vi "Serial Write and Read on Two Ports 4.0.vi"(10 "VISA Resource (write)":refnum<visa-resource-name>="COM5", 11 "Write String":string="DPOS=5000") -> (3 "Read String":string="EPOS=2\n")   [LabVIEW 2019]
doc: "This example opens two VISA resources and configures one COM port to perform a write operation and the other COM port to perform a read operation. This VI will wait until the specified number of bytes is received at the port or until a termination character is read.\n\nThis example allows you perform diagnostic tests on your ports. You can use this example to perform a wrap-back test. Both serial ports must have the same basic configuration parameters. You can connect two of the ports using a null modem cable, which effectively connects one port's RX lines to the other port's TX lines. If you use a straight-through cable, one port's RX lines will be connected to the other port's RX lines, and you cannot communicate between the two ports."
uses:
  Program Files (x86)/National Instruments/LabVIEW 2019/instr.lib/LPT/LPT-GUI-MIC-ver 4 Randy Folder/examples/Instrument IO/Serial/support/Serial - Settings.ctl
  <vilib>/Instr/_visa.llb/VISA Configure Serial Port (Instr).vi
panel:
  in  "Serial Settings (read)":T1={"baud rate"=9600, "data bits"=8, "parity"=enum."None", "stop bits"=10, "flow control"=0} {"flow control" items=["None"=0, "XON/XOFF"=1, "RTS/CTS"=2, "DTR/DSR"=4]; "stop bits" items=["1.0"=10, "1.5"=15, "2.0"=20]; "data bits" min=5 max=8 step=1; "baud rate" items=["75"=75, "110"=110, "134"=134, "150"=150, "300"=300, "600"=600, "1200"=1200, "1800"=1800, "2400"=2400, "4800"=4800, "7200"=7200, "9600"=9600, "14400"=14400, "19200"=19200, "28800"=28800, "38400"=38400, "56000"=56000, "57600"=57600, "115200"=115200, "128000"=128000, "230400"=230400]}
  in  "Serial Settings (write)":T1={"baud rate"=9600, "data bits"=8, "parity"=enum."None", "stop bits"=10, "flow control"=0} {"flow control" items=["None"=0, "XON/XOFF"=1, "RTS/CTS"=2, "DTR/DSR"=4]; "stop bits" items=["1.0"=10, "1.5"=15, "2.0"=20]; "data bits" min=5 max=8 step=1; "baud rate" items=["75"=75, "110"=110, "134"=134, "150"=150, "300"=300, "600"=600, "1200"=1200, "1800"=1800, "2400"=2400, "4800"=4800, "7200"=7200, "9600"=9600, "14400"=14400, "19200"=19200, "28800"=28800, "38400"=38400, "56000"=56000, "57600"=57600, "115200"=115200, "128000"=128000, "230400"=230400]}
  out "bytes read":u32=7
  out "VISA Resource (read)":refnum<visa-resource-name>="COM5"
  out "bytes written":u32=9
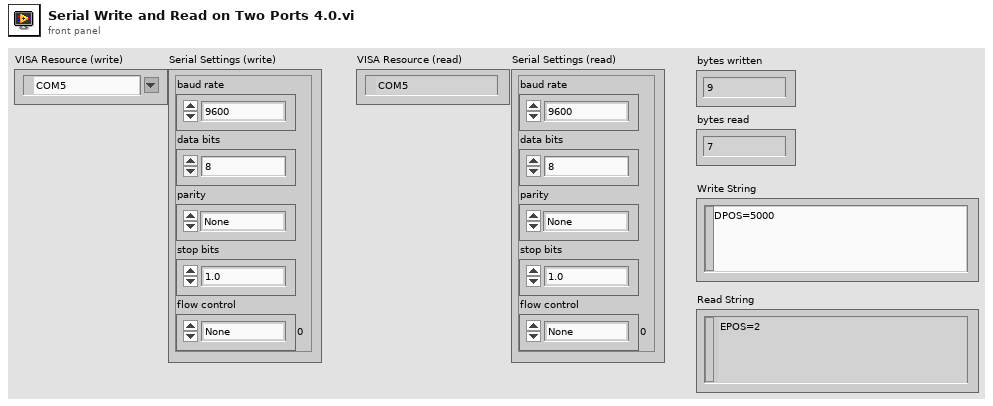
[diagram p1: front panel]
types:
  T1 = typedef "Serial - Settings.ctl" = cluster{"baud rate":u32, "data bits":u16, "parity":enum16{"None", "Odd", "Even", "Mark", "Space"}, "stop bits":u16, "flow control":u16}
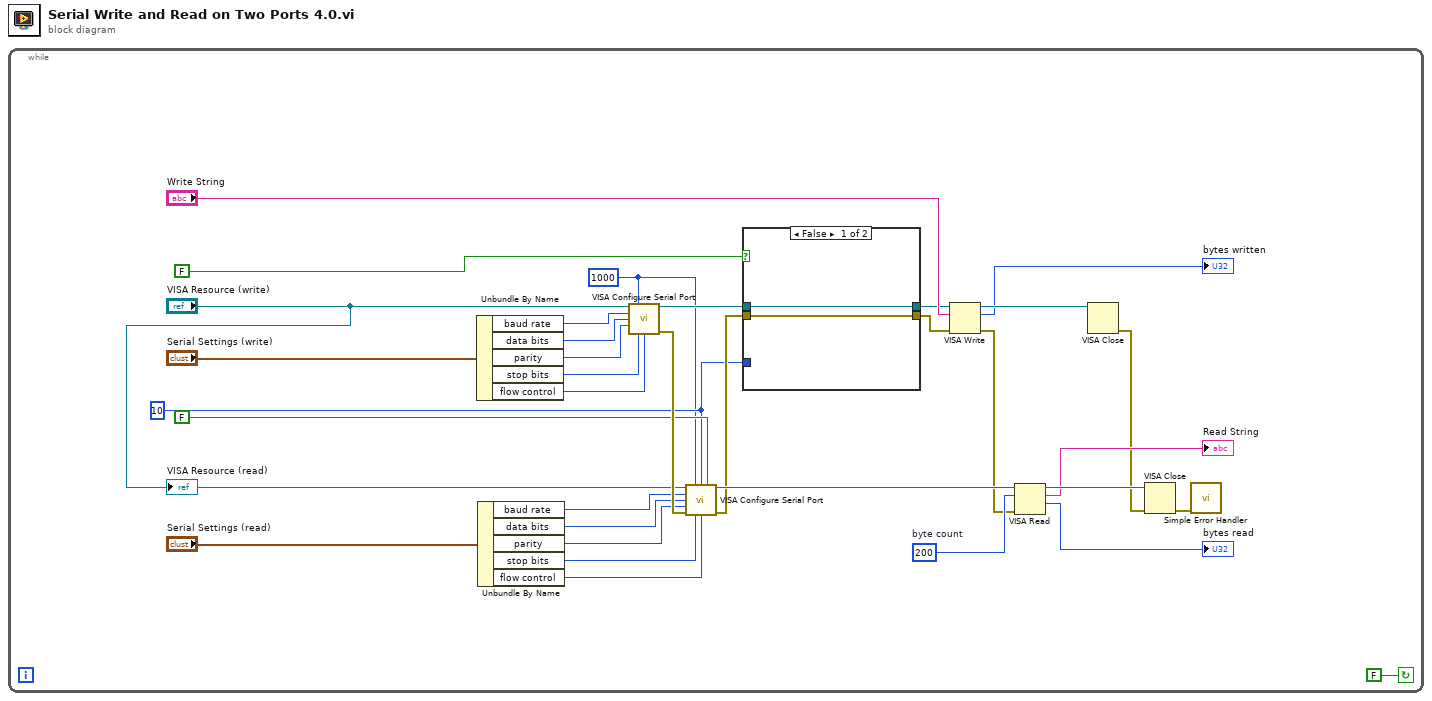
[diagram p0: block diagram]
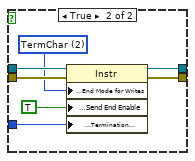
[diagram p2: hidden frame]
diagram:
  n1 = while {
    stop <- FALSE continue-if-true
    w4 = u8 10 ("Termination Character")
    w3 = u32 1000 ("timeout (10sec)")
    w29 = u32 200  # byte count
    n2 = Unbundle By Name("Serial Settings (write)") -> ("baud rate"=w22:u32, "data bits"=w21:u16, "parity"=w20:enum16{"None", "Odd", "Even", "Mark", "Space"}, "stop bits"=w19:u16, "flow control"=w18:u16)
    n3 = Unbundle By Name("Serial Settings (read)") -> ("baud rate"=w16:u32, "data bits"=w15:u16, "parity"=w14:enum16{"None", "Odd", "Even", "Mark", "Space"}, "stop bits"=w13:u16, "flow control"=w12:u16)
    n4 = call-poly "VISA Configure Serial Port"("VISA resource name"="VISA Resource (write)", "timeout (10sec)"=w3, "baud rate (9600)"=w22, "data bits (8)"=w21, "parity (0:none)"=w20, "stop bits (10: 1 bit)"=w19, "flow control (0:none)"=w18) -> ("VISA resource name out"=w9:refnum<visa-resource-name>, "error out"=w27:errorcluster)  [unwired: 2 in, 5 out]
    n5 = call-poly "VISA Configure Serial Port"("VISA resource name"="VISA Resource (write)", "timeout (10sec)"=w3, "termination char\n(0xA = '\\n' = LF)"=w4, "Enable Termination\nChar (T)"=FALSE ("End Read on Termination Character?"), "baud rate (9600)"=w16, "data bits (8)"=w15, "parity (0:none)"=w14, "error in (no error)"=w27, "stop bits (10: 1 bit)"=w13, "flow control (0:none)"=w12) -> ("VISA resource name out"=w33:refnum<visa-resource-name>, "error out"=w7:errorcluster)  [unwired: 4 out]
    n6 = case shown="False" FALSE ("End Write on Termination Character?") {
      tunnel: w9 -> [w35 w43]
      tunnel: w7 -> [w36 w42]
      tunnel: [w35 w41] -> w8
      tunnel: [w36 w40] -> w6
      tunnel: w4 -> [_ w38]
      frame False {
      }
      frame True {
        w39 = u16 2 items=["None", "LastBit", "TermChar", "Break"] ("Serial Settings:Serial End Mode for Writes")
        n7 = property class="Instr"(reference=w43, error in=w42, "Serial Settings:End Mode for Writes"=w39, "Message Based Settings:Send End Enable"=TRUE, "Message Based Settings:Termination Character"=w38) -> (reference out=w41:refnum<visa-resource-name>, error out=w40:errorcluster)
      }
    }
    n8 = VISA Write(VISA resource name=w8, write buffer="Write String", error in (no error)=w6) -> (VISA resource name out=w34:refnum<visa-resource-name>, return count=→"bytes written":u32, error out=w26:errorcluster)
    n9 = VISA Read(VISA resource name=w33, byte count=w29, error in (no error)=w26) -> (VISA resource name out=w32:refnum<visa-resource-name>, read buffer=→"Read String":string, return count=→"bytes read":u32)  [unwired: 1 out]
    n10 = VISA Close(VISA resource name=w34) -> (error out=w25:errorcluster)  [unwired: 1 in]
    n11 = VISA Close(VISA resource name=w32, error in (no error)=w25) -> (error out=w24:errorcluster)
    n12 = call <vilib>:"Simple Error Handler.vi"("error in (no error)"=w24) -> ()  [unwired: 1 in, 8 out]
    "VISA Resource (read)" <- "VISA Resource (write)"
  }
